vi "Start Sync.vi"(8 "error in (no error)":errorcluster, 11 "gRPC Server in":refnum<class "veristand-grpc.lvclass">) -> (0 "error out":errorcluster, 3 "gRPC Server out":refnum<class "veristand-grpc.lvclass">)   [LabVIEW 2020, in "Veristandgrpc_server.lvlib" / "veristand-grpc.lvclass"]
uses:
  veristand-grpc.lvclass
  veristand-grpc.lvclass/veristand-grpc.ctl
  RPC Messages/Get veristand_Request.vi
  Data/Write.vi
  RPC Messages/Set veristand_Reponse.vi
  Data/Read.vi
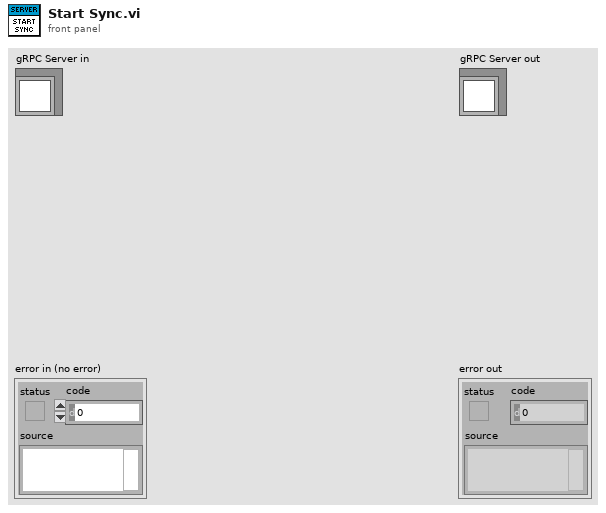
[diagram p1: front panel]
types:
  T1 = typedef "Veristandgrpc_server.lvlib/veristand-grpc.lvclass/Server Internal UEs.ctl" = cluster{"veristand Write Internal UE":refnum<user-event>, "veristand Read Internal UE":refnum<user-event>}
  T2 = typedef "Veristandgrpc_server.lvlib/veristand-grpc.lvclass/Server gRPC UEs.ctl" = cluster{"veristand Write gRPC UE":refnum<user-event>, "veristand Read gRPC UE":refnum<user-event>}
  T3 = typedef "grpc-lvsupport-release.lvlib/grpcId.ctl" = u64
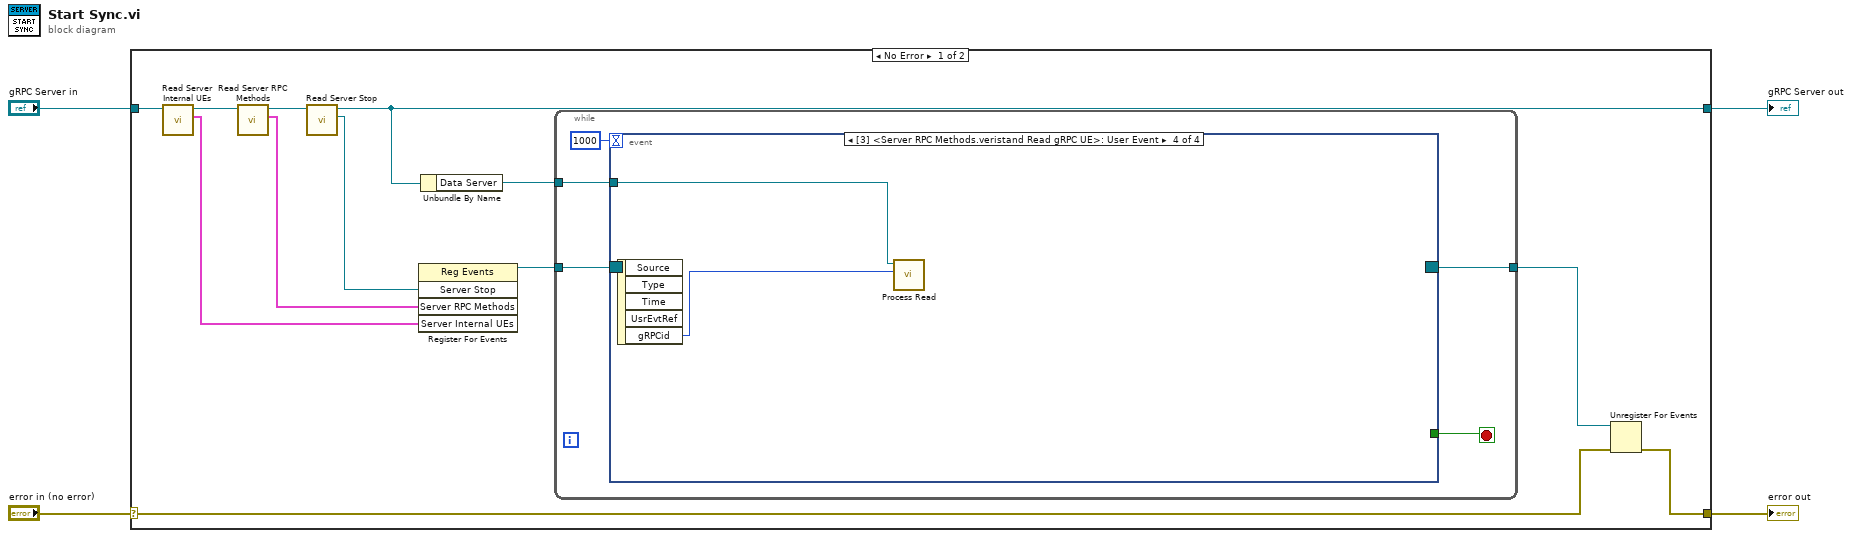
[diagram p0: block diagram]
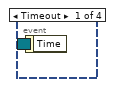
[diagram p2: hidden frame]
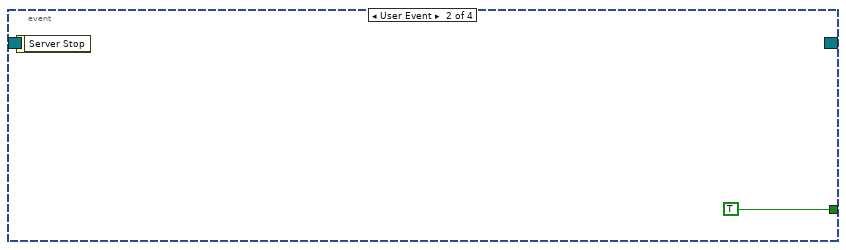
[diagram p3: hidden frame]
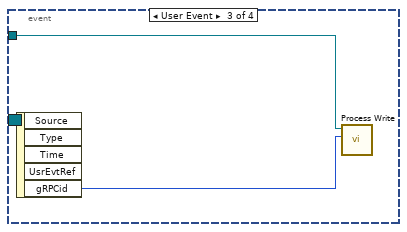
[diagram p4: hidden frame]
diagram:
  n1 = case shown="No Error" "error in (no error)" {
    selector: "error in (no error)" -> [w10 w28]
    tunnel: [w9 w28] -> w3
    tunnel: [w6 w27] -> w1
    tunnel: "gRPC Server in" -> [w16 w27]
    frame No Error {
      n2 = call "Read Server Internal UEs.vi"("SignalGeneratorService in"=w16) -> ("Server Internal UEs"=w14:T1, "SignalGeneratorService out"=w15:refnum<class "veristand-grpc.lvclass">)  [unwired: 8 in, 1 out]
      n3 = call "Read Server RPC Methods.vi"("SignalGeneratorService in"=w15) -> ("Server RPC Methods"=w8:T2, "SignalGeneratorService out"=w13:refnum<class "veristand-grpc.lvclass">)  [unwired: 8 in, 1 out]
      n4 = call-dynamic "Read Server Stop.vi"("iService in"=w13) -> ("Server Stop"=w7:refnum<user-event>, "iService out"=w6:refnum<class "veristand-grpc.lvclass">)  [unwired: 8 in, 1 out]
      n5 = register-events(w7, w8, w14) -> (reference out=w12:refnum<event-registration>)  [unwired: 2 in, 1 out]
      n6 = Unbundle By Name(w6) -> ("Data Server"=w5:refnum<class "Data Server.lvclass">)
      n7 = while {
        tunnel: w12 -> [w21]
        tunnel: [w19] -> w11
        tunnel: w5 -> [w17]
        stop <- w20 stop-if-true
        n8 = event "RPC Methods Event Structure" shown="[3] <Server RPC Methods.veristand Read gRPC UE>: User Event" {
          selector: w21 -> [_ _ _ _]
          dyn-events: [_ _ _ _] -> w19
          timeout: 1000 -> [_ _ _ _]
          tunnel: [_ TRUE _ _] -> w20
          tunnel: w17 -> [_ _ w24 w26]
          event Timeout {
            n9 = event-data() -> ()  [unwired: 1 in, 1 out]
          }
          event User Event {
            n10 = event-data() -> ()  [unwired: 1 in, 1 out]
          }
          event User Event {
            n11 = event-data() -> ("gRPCid"=w23:T3)  [unwired: 1 in, 4 out]
            n12 = call "Process Write.vi"("gRPCid"=w23, "Data Server"=w24) -> ()  [unwired: 9 in, 1 out]
          }
          event User Event {
            n13 = event-data() -> ("gRPCid"=w25:T3)  [unwired: 1 in, 4 out]
            n14 = call "Process Read.vi"("gRPCid"=w25, "Data Server"=w26) -> ()  [unwired: 9 in, 1 out]
          }
        }
      }
      n15 = Unregister For Events(event registration refnum=w11, error in=w10) -> (error out=w9:errorcluster)
    }
    frame Error {
    }
  }
  "error out" <- w3
  "gRPC Server out" <- w1
